vi "Load Face.vi"(8 "error in (no error)":errorcluster, 10 "Font Path":path, 11 "Freetype Drawer in":refnum<class "Freetype Drawer.lvclass">) -> (0 "error out":errorcluster, 2 "face ref":i64, 3 "Freetype Drawer out":refnum<class "Freetype Drawer.lvclass">)   [LabVIEW 2023, in "Freetype Drawer.lvlib" / "Freetype Drawer.lvclass"]
uses:
  Freetype Drawer.lvclass
  Freetype Drawer.lvclass/Freetype Drawer.ctl
  <vilib>/Utility/miscctls.llb/LVMapReplaceAction.ctl
  Freetype Drawer.lvlib
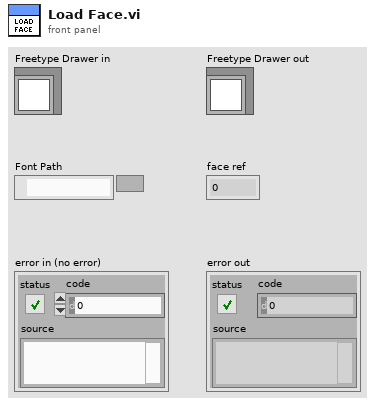
[diagram p1: front panel]
types:
  T1 = typedef "LVMapReplaceAction.ctl" = enum32{"Modify Entry only if found", "Add or Modify Entry", "Delete Entry"}
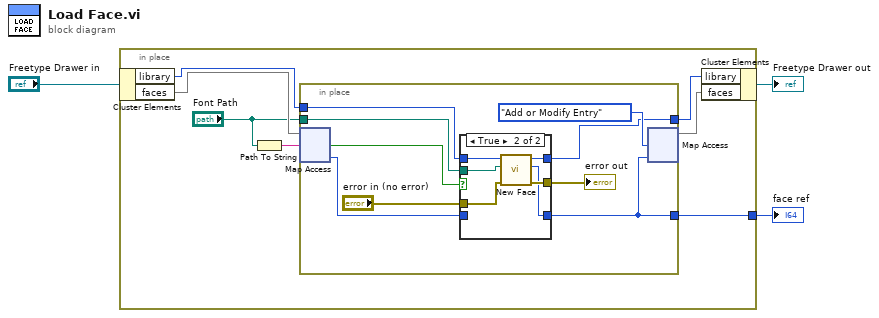
[diagram p0: block diagram]
diagram:
  n1 = in-place {
    in-place-border: [w9] -> w3
    n2 = in-place-cluster #1("Freetype Drawer in") -> ("library"=w7:i64, "faces"=w10:map{string, i64})
    n3 = Path To String(path="Font Path") -> (string=w5:string)
    n4 = in-place {
      in-place-border: "Font Path" -> [w19]
      in-place-border: [w16] -> w9
      in-place-border: w7 -> [w14]
      in-place-border: [w13] -> w6
      n5 = in-place-map #2(w10, w5) -> (w15:i64, w18:bool)  [unwired: 1 in]
      n6 = case shown="True" w18 {
        tunnel: [w21 w28] -> w11
        tunnel: [w22 w27] -> w16
        tunnel: w14 -> [w20 w26]
        tunnel: "error in (no error)" -> [w21 w25]
        tunnel: w19 -> [_ w24]
        tunnel: w15 -> [w22 _]
        tunnel: [w20 w23] -> w13
        frame False {
        }
        frame True {
          n7 = call "New Face.vi"("error in (no error)"=w25, "Path"=w24, "library in"=w26) -> ("error out"=w28:errorcluster, "face out"=w27:i64, "library out"=w23:i64)  [unwired: 6 in]
        }
      }
      "error out" <- w11
      n8 = in-place-map #2(w16, LVMapReplaceAction."Add or Modify Entry" ("action")) -> (w8:map{string, i64})  [unwired: 2 out]
    }
    n9 = in-place-cluster #1("library"=w6, "faces"=w8) -> (→"Freetype Drawer out":refnum<class "Freetype Drawer.lvclass">)
  }
  "face ref" <- w3
